vi "DatabaseAPI-Insert.vi"(7 "Cluster Data for DB":variant, 8 "error in (no error)":errorcluster, 10 "Table":string, 11 "Database-API in":refnum<class "Database-API.lvclass">) -> (0 "error out":errorcluster, 3 "Database-API out":refnum<class "Database-API.lvclass">)   [LabVIEW 2014, in "Database-API.lvclass"]
uses:
  Database-API.lvclass
  Database-API.lvclass/Database-API.ctl
  <vilib>/addons/database/NI_Database_API.lvlib
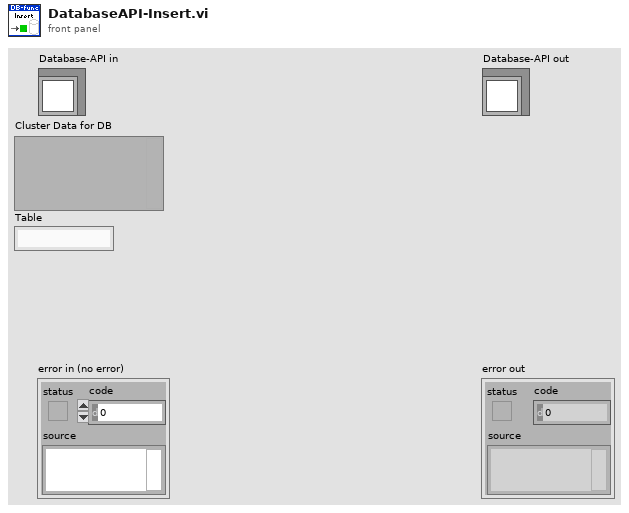
[diagram p1: front panel]
types:
  T1 = typedef "NI_Database_API.lvlib/Conn ObjectReference.ctl" = refnum<k1>
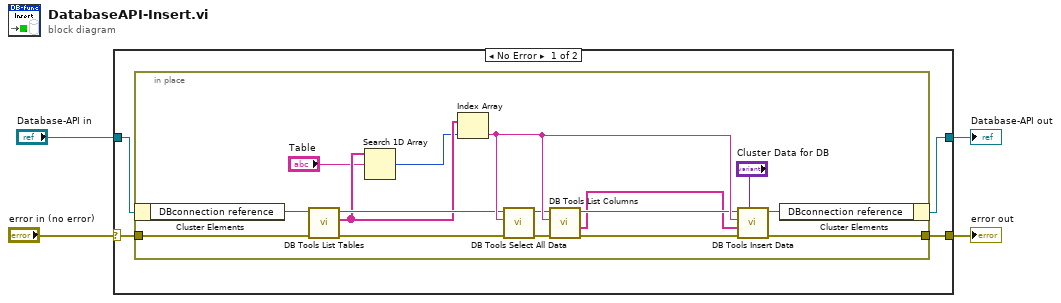
[diagram p0: block diagram]
diagram:
  n1 = case shown="No Error" "error in (no error)" {
    selector: "error in (no error)" -> [w8 w26]
    tunnel: [w6 w26] -> w3
    tunnel: [w5 w25] -> w1
    tunnel: "Database-API in" -> [w7 w25]
    frame No Error {
      n2 = in-place {
        in-place-border: w8 -> [w16]
        in-place-border: [w12] -> w6
        n3 = in-place-cluster #1(w7) -> ("DBconnection reference"=w15:T1)
        n4 = call <vilib>:"DB Tools List Tables.vi"("error in (no error)"=w16, "connection reference"=w15) -> ("error out"=w20:errorcluster, "tables"=w11:string[], "connection reference out"=w18:T1)  [unwired: 3 in]
        n5 = Search 1D Array(1D array=w11, element="Table") -> (index of element=w9:i32)  [unwired: 1 in]
        n6 = Index Array(array=w11, index=w9) -> (element=w24:string)
        n7 = call <vilib>:"DB Tools Select All Data.vi"("error in (no error)"=w20, "table"=w24, "connection reference"=w18) -> ("error out"=w19:errorcluster, "connection reference out"=w17:T1)  [unwired: 3 in, 1 out]
        n8 = call <vilib>:"DB Tools List Columns.vi"("error in (no error)"=w19, "table"=w24, "connection reference"=w17) -> ("error out"=w21:errorcluster, "columns"=w22:string[], "connection reference out"=w23:T1)  [unwired: 1 in, 1 out]
        n9 = call <vilib>:"DB Tools Insert Data.vi"("data"="Cluster Data for DB", "error in (no error)"=w21, "columns"=w22, "table"=w24, "connection reference"=w23) -> ("error out"=w12:errorcluster, "connection reference out"=w14:T1)  [unwired: 5 in]
        n10 = in-place-cluster #1("DBconnection reference"=w14) -> (w5:refnum<class "Database-API.lvclass">)
      }
    }
    frame Error {
    }
  }
  "error out" <- w3
  "Database-API out" <- w1
